vi "Video Stream Client Host.vi"(10 "Close ref":refnum<vi>, 11 "occurrence":refnum<k4>) -> ()   [LabVIEW 2015]
uses:
  RT Controls/Generic instruction typedef.ctl
  <vilib>/vision/Image Controls.llb/IMAQ Image.ctl
  IP Dev Area/IP results.ctl
  Robo Team Globals.vi
  GUI/Host Globals.vi
  <resource>/objmgr/ni.dex.rc
panel:
  out "Frame Rate":dbl
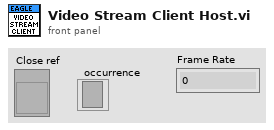
[diagram p1: front panel]
types:
  T1 = typedef "Image Type" = u32
  T2 = typedef "IMAQ Image.ctl" = refnum<image>
  T3 = typedef "Generic instruction typedef.ctl" = cluster{"CMD":string, "Data":variant}
  T4 = typedef "IP results.ctl" = cluster{"X":u16, "Y":u16, "A":dbl, "B":dbl, "Grade":u16, "Frame#":u16}
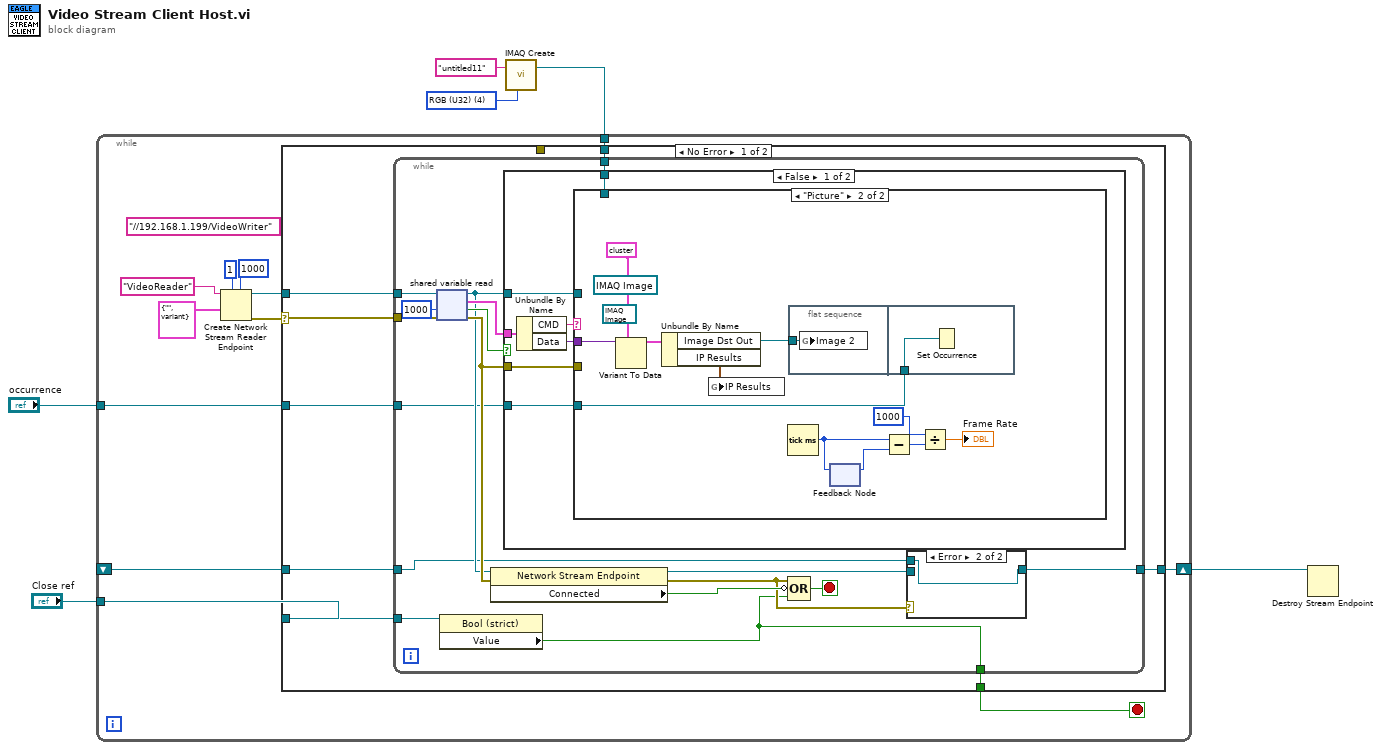
[diagram p0: block diagram]
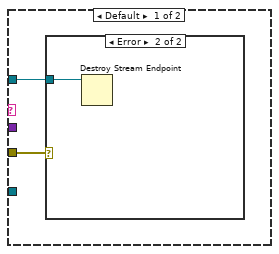
[diagram p3: hidden frame]
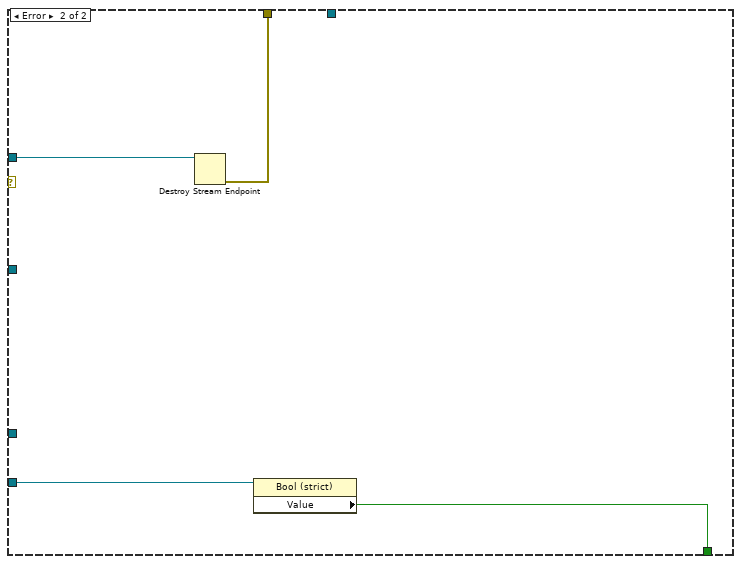
[diagram p6: hidden frame]
diagram:
  w2 = T1 4 items=["Grayscale (U8)", "Grayscale (I16)", "Grayscale (SGL)", "Complex (CSG)", "RGB (U32)", "HSL (U32)", "RGB (U64)", "Grayscale (U16)"] ("Image Type")
  n1 = call "IMAQ Create"("Image Name"="untitled11", "Image Type"=w2) -> ("New Image"=w1:T2)  [unwired: 3 in, 1 out]
  n2 = while {
    shift-right: [w11] -> w4
    shift-left: _ -> [w10]
    tunnel: "occurrence" -> [w9]
    tunnel: "Close ref" -> [w8]
    tunnel: w1 -> [w7]
    stop <- w13 stop-if-true
    (unwired) "//192.168.1.199/VideoWriter" ("writer url")
    n3 = Create Network Stream Reader Endpoint(5:1000 ("timeout in ms (-1)"), 7:1 ("reader buffer size"), 9:T3 {"CMD"="", "Data"=variant}, 11:"VideoReader" ("name (unnamed)")) -> (0:w12:errorcluster, 3:w16:refnum<k21>)  [unwired: 3 in]
    n4 = case shown="No Error" w12 {
      selector: w12 -> [w21 _]
      tunnel: w16 -> [w26 w71]
      tunnel: [w25 w69] -> w13
      tunnel: [w24 _] -> w11
      tunnel: w10 -> [w23 _]
      tunnel: w9 -> [w22 _]
      tunnel: [_ w72] -> _
      tunnel: w8 -> [w20 w70]
      tunnel: w7 -> [w19 _]
      frame No Error {
        n5 = while {
          tunnel: w26 -> [w40]
          tunnel: [w29] -> w25
          tunnel: [w33] -> w24
          tunnel: w23 -> [w32]
          tunnel: w22 -> [w31]
          tunnel: w21 -> [w30]
          tunnel: w20 -> [w28]
          tunnel: w19 -> [w27]
          stop <- w41 stop-if-true
          n6 = shared-variable-read(w40, w30, 1000 ("timeout ms (-1)")) -> (w36:refnum<k21>, w38:errorcluster, w42:bool, w43:T3)
          n7 = property class="Bool (strict)"(reference=w28) -> ("Value"=w29:bool)  [unwired: 1 in, 2 out]
          n8 = property class="Network Stream Endpoint"(reference=w36, error in=w38) -> (reference out=w34:refnum<k21>, error out=w35:errorcluster, "Connected"=w37:bool)
          n9 = case shown="False" w42 {
            tunnel: w43 -> [w52 _]
            tunnel: w38 -> [w49 _]
            tunnel: w36 -> [w48 _]
            tunnel: w31 -> [w47 _]
            tunnel: w27 -> [w46 _]
            frame False {
              n10 = Unbundle By Name(w52) -> ("CMD"=w51:string, "Data"=w50:variant)
              n11 = case shown="\"Picture\"" w51 {
                tunnel: w50 -> [_ w66]
                tunnel: w49 -> [w54 _]
                tunnel: w48 -> [w53 _]
                tunnel: w47 -> [_ w65]
                tunnel: w46 -> [_ _]
                frame Default {
                  n12 = case shown="Error" w54 {
                    tunnel: w53 -> [_ w55]
                    frame No Error {
                    }
                    frame Error {
                      n13 = Destroy Stream Endpoint(11:w55) -> ()  [unwired: 1 in, 1 out]
                    }
                  }
                }
                frame "Picture" {
                  (unwired) T2 refnum ("Image")
                  (unwired) T2 refnum ("Image")
                  n14 = Variant To Data(type=cluster{"Image Dst Out":T2, "IP Results":T4} {"Image Dst Out"=refnum, "IP Results"={"X"=0, "Y"=0, "A"=0.0, "B"=0.0, "Grade"=0, "Frame#"=0}} ("output cluster"), Variant=w66) -> (data=w57:cluster{"Image Dst Out":T2, "IP Results":T4})  [unwired: 1 in, 1 out]
                  n15 = Unbundle By Name(w57) -> ("Image Dst Out"=w59:T2, "IP Results"=w58:T4)
                  n16 = global write "Robo Team Globals.vi" "IP Results"(w58) -> ()
                  n17 = Tick Count (ms)() -> (millisecond timer value=w64:u32)
                  n18 = flat-sequence {
                    tunnel: w59 -> [w67]
                    tunnel: w65 -> [w68]
                    frame #0 {
                      n19 = global write "Host Globals.vi" "Image 2"(w67) -> ()
                    }
                    frame #1 {
                      n20 = Set Occurrence(w68) -> ()
                    }
                  }
                  n21 = feedback-in #1(w64) -> ()
                  n22 = feedback #1() -> (w63:u32)  [unwired: 1 in]
                  n23 = Subtract(x=w64, y=w63) -> (x-y=w62:u32)
                  n24 = Divide(x=u32 1000, y=w62) -> (x/y=→"Frame Rate":dbl)
                }
              }
            }
            frame True {
            }
          }
          n25 = Compound Arithmetic op=OR(w35, invert w37, w29) -> (w41:bool)
          n26 = case shown="Error" w35 {
            tunnel: [w44 w45] -> w33
            tunnel: w34 -> [w44 _]
            tunnel: w32 -> [_ w45]
            frame No Error {
            }
            frame Error {
            }
          }
        }
      }
      frame Error {
        n27 = Destroy Stream Endpoint(11:w71) -> (0:w72:errorcluster)  [unwired: 1 in]
        n28 = property class="Bool (strict)"(reference=w70) -> ("Value"=w69:bool)  [unwired: 1 in, 2 out]
      }
    }
  }
  n29 = Destroy Stream Endpoint(11:w4) -> ()  [unwired: 1 in, 1 out]
